vi "ReadWrite.Initialize.vi"(8 "error in (no error)":errorcluster, 11 "Settings":T2 {"Refs" format="%.0x"}) -> (0 "error out":errorcluster, 3 "ReadWrite out":refnum<class "ReadWrite.lvclass">)   [LabVIEW 2023, in "Data Access Engine.lvlib" / "ReadWrite.lvclass"]
uses:
  ReadWrite.lvclass
  ReadWrite.lvclass/ReadWrite.ctl
  <vilib>/NI VeriStand/Custom Device API/Data Reference.ctl
  <vilib>/NI VeriStand/Custom Device API/Custom Device API.lvlib
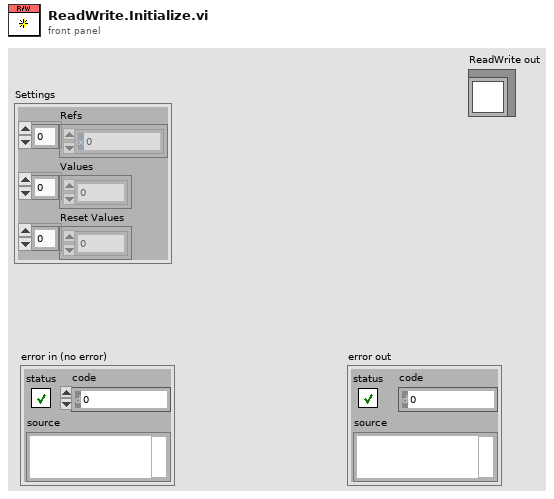
[diagram p1: front panel]
types:
  T1 = typedef "Custom Device API.lvlib/Data Reference.ctl" = i32
  T2 = cluster{"Refs":T1[], "Values":dbl[], "Reset Values":dbl[]}
  T3 = cluster{"read mode":enum16{"polling", "blocking"}, "write mode":enum16{"polling", "blocking"}}
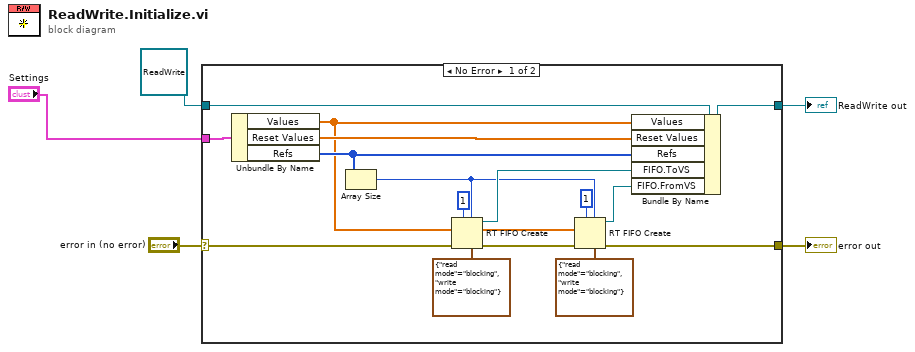
[diagram p0: block diagram]
diagram:
  n1 = case shown="No Error" "error in (no error)" {
    selector: "error in (no error)" -> [w10 w23]
    tunnel: [w15 w23] -> w5
    tunnel: refnum<class "ReadWrite.lvclass"> refnum ("ReadWrite in") -> [w12 w22]
    tunnel: [w11 w22] -> w3
    tunnel: "Settings" -> [w9 _]
    frame No Error {
      n2 = Unbundle By Name(w9) -> ("Values"=w6:dbl[], "Reset Values"=w7:dbl[], "Refs"=w8:T1[])
      n3 = Array Size(array=w8) -> (size(s)=w14:i32)
      n4 = RT FIFO Create(1:w6, 3:w10, 4:u32 1 ("size (10)"), 6:w14, 7:T3 {"read mode"=enum."blocking", "write mode"=enum."blocking"} ("r/w modes (polling,polling)")) -> (8:w20:refnum<k33>, 11:w13:errorcluster)  [unwired: 3 in, 1 out]
      n5 = RT FIFO Create(1:w6, 3:w13, 4:u32 1 ("size (10)"), 6:w14, 7:T3 {"read mode"=enum."blocking", "write mode"=enum."blocking"} ("r/w modes (polling,polling)")) -> (8:w21:refnum<k33>, 11:w15:errorcluster)  [unwired: 3 in, 1 out]
      n6 = Bundle By Name(cluster=w12, "Values"=w6, "Reset Values"=w7, "Refs"=w8, "FIFO.ToVS"=w20, "FIFO.FromVS"=w21) -> (w11:refnum<class "ReadWrite.lvclass">)
    }
    frame Error {
    }
  }
  "error out" <- w5
  "ReadWrite out" <- w3
